vi "Erase_Pixel_at_Coords.vi"(8 "y-axis":dbl, 9 "x-axis":dbl, 11 "Input array":bool[][](array[boolean])) -> (3 "Ouput array":bool[][](array[boolean]))   [LabVIEW 2015]
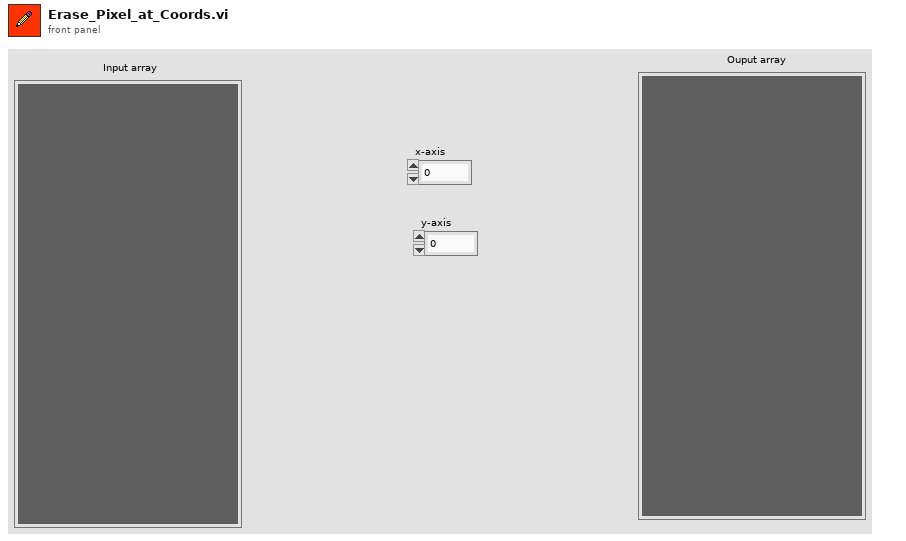
[diagram p1: front panel]
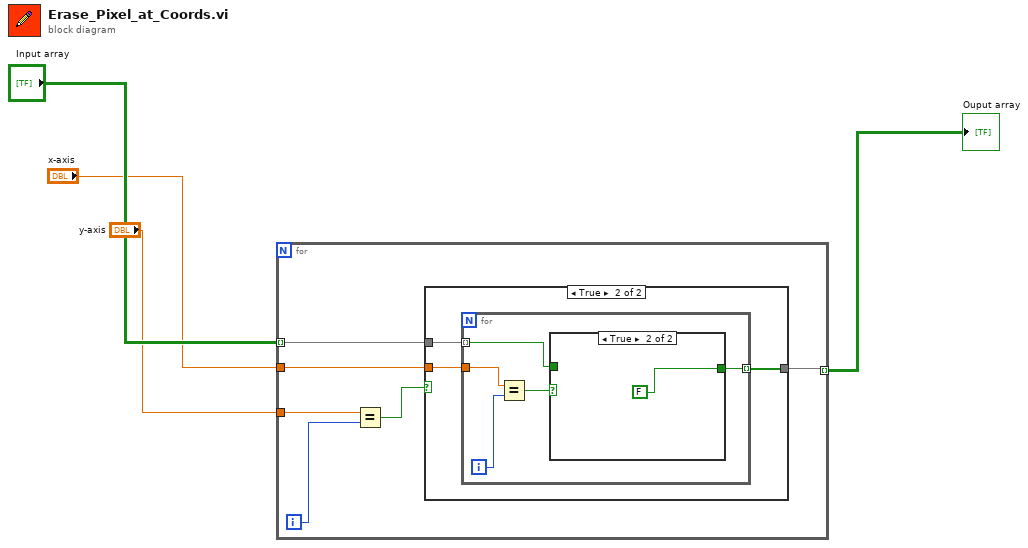
[diagram p0: block diagram]
diagram:
  n1 = for {
    tunnel: "y-axis" -> [w8]
    tunnel: "x-axis" -> [w7]
    tunnel: "Input array" -> [w6] mode=indexing
    tunnel: [w5] -> w4 mode=indexing
    i -> [w10]
    n2 = Equal?(x=w8, y=w10) -> (x = y?=w9:bool)
    n3 = case shown="True" w9 {
      tunnel: w7 -> [_ w14]
      tunnel: w6 -> [w11 w13]
      tunnel: [w11 w12] -> w5
      frame False {
      }
      frame True {
        n4 = for {
          tunnel: w14 -> [w17]
          tunnel: w13 -> [w16] mode=indexing
          tunnel: [w15] -> w12 mode=indexing
          i -> [w18]
          n5 = Equal?(x=w17, y=w18) -> (x = y?=w19:bool)
          n6 = case shown="True" w19 {
            tunnel: w16 -> [w20 _]
            tunnel: [w20 FALSE] -> w15
            frame False {
            }
            frame True {
            }
          }
        }
      }
    }
  }
  "Ouput array" <- w4
